vi "To String and From String Array Test.vi"() -> ()   [LabVIEW 2015, in "Wait On Boolean Tests.lvlib"]
uses:
  Wait On Boolean Tests.lvlib
  <vilib>/NI/Tag Bus/tag/Data Type.ctl
  <vilib>/NI/Tag Bus Module Framework/channel/channel classification.ctl
  Config/Wait On Boolean Step Config.lvclass
  Config/Wait On Boolean Step Config.lvclass/Wait On Boolean Step Config.ctl
  Config/Write Wait On Boolean Event.vi
  <vilib>/NI/Tag Bus/tag/tag descriptor.lvclass
  <vilib>/NI/Tag Bus Module Framework/channel/TBM channel.lvclass
panel:
  out "Pass?":bool
  out "error out":errorcluster
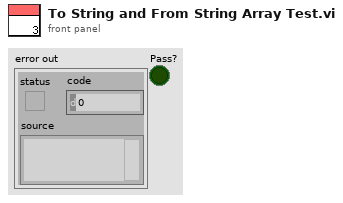
[diagram p1: front panel]
types:
  T1 = typedef "TBM channel.lvclass/channel classification.ctl" = enum16{"input data", "output data", "processing parameter", "processing result"}
  T2 = typedef "tag bus.lvlib/tag descriptor.lvclass/Data Type.ctl" = enum16{"Double", "Single", "I64", "I32", "I16", "I8", "U64", "U32", "U16", "U8", "Boolean", "String", "Array of Double", "Array of Single", "Array of I64", "Array of I32", "Array of I16", "Array of I8", "Array of U64", "Array of U32", "Array of U16", "Array of U8", "Array of Boolean", "Array of String"}
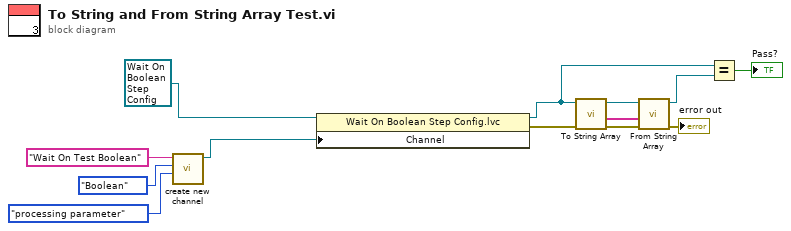
[diagram p0: block diagram]
diagram:
  n1 = call <vilib>:"create new channel.vi"("channel classification"=channel_classification."processing parameter", "data type"=Data_Type."Boolean" ("Data Type"), "channel name"="Wait On Test Boolean" ("Jump Tag Name")) -> ("channel"=w9:refnum<class "TBM channel.lvclass">)  [unwired: 8 in]
  n2 = property class="Wait On Boolean Step Config.lvc"(reference=refnum<class "Wait On Boolean Step Config.lvclass"> refnum ("Wait On Boolean Step Config.lvclass"), "Channel"=w9) -> (reference out=w6:refnum<class "Wait On Boolean Step Config.lvclass">, error out=w8:errorcluster)  [unwired: 1 in]
  n3 = call-dynamic "To String Array.vi"("error in (no error)"=w8, "Wait On Boolean Config in"=w6) -> ("error out"=w7:errorcluster, "Step String Array"=w1:string[], "Wait On Boolean Config out"=w5:refnum<class "Wait On Boolean Step Config.lvclass">)  [unwired: 7 in]
  n4 = call-dynamic "From String Array.vi"("error in (no error)"=w7, "String Array"=w1, "Wait On Boolean Config in"=w5) -> ("error out"=→"error out":errorcluster, "Wait On Boolean Config out"=w4:refnum<class "Wait On Boolean Step Config.lvclass">)  [unwired: 6 in, 1 out]
  n5 = Equal?(x=w6, y=w4) -> (x = y?=→"Pass?":bool)
